vi "line to strings.vi"(11 "line":T1) -> (3 "strings":string[](array[string]))   [LabVIEW 2013, in "EthernetIP editor node.lvclass"]
uses:
  EthernetIP editor node.lvclass
  table line.ctl
  <vilib>/NI/TBM Modules/Ethernet IP/channel/EthernetIP Channel.lvclass
  <vilib>/NI/Tag Bus/tag/tag descriptor.lvclass/tag descriptor.ctl
  <vilib>/NI/TBM Modules/Ethernet IP/channel/EthernetIP Channel.lvclass/EthernetIP Channel.ctl
  <vilib>/NI/Tag Bus Module Framework/channel/TBM channel.lvclass/TBM channel.ctl
  <vilib>/NI/Tag Bus/tag/read tag name.vi
  <vilib>/NI/TBM Modules/Ethernet IP/channel/Read Instance ID.vi
  <vilib>/NI/Tag Bus Module Framework/channel/Read channel classification.vi
  <vilib>/NI/TBM Modules/Ethernet IP/channel/Read byte index.vi
  <vilib>/NI/TBM Modules/Ethernet IP/channel/Read subindex.vi
  <vilib>/NI/Tag Bus/tag/read data type.vi
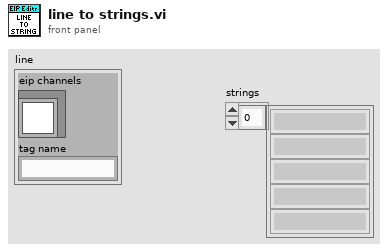
[diagram p1: front panel]
types:
  T1 = typedef "EthernetIP editor node.lvclass/table line.ctl" = cluster{"eip channels":refnum<class "EthernetIP Channel.lvclass">, "tag name":string}
  T2 = typedef "TBM channel.lvclass/channel classification.ctl" = enum16{"input data", "output data", "processing parameter", "processing result"}
  T3 = typedef "tag bus.lvlib/tag descriptor.lvclass/Data Type.ctl" = enum16{"Double", "Single", "I64", "I32", "I16", "I8", "U64", "U32", "U16", "U8", "Boolean", "String", "Array of Double", "Array of Single", "Array of I64", "Array of I32", "Array of I16", "Array of I8", "Array of U64", "Array of U32", "Array of U16", "Array of U8", "Array of Boolean", "Array of String"}
  T4 = typedef "EthernetIP configuration.lvclass/assembly type.ctl" = enum32{"Producing", "Consuming"}
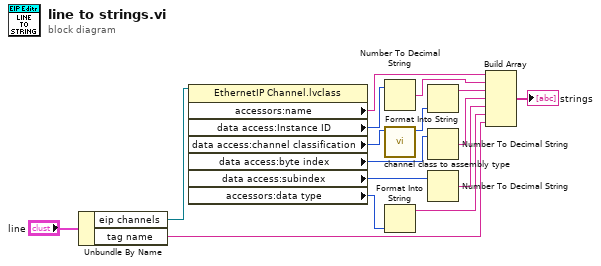
[diagram p0: block diagram]
diagram:
  n1 = Unbundle By Name("line") -> ("eip channels"=w11:refnum<class "EthernetIP Channel.lvclass">, "tag name"=w14:string)
  n2 = property class="EthernetIP Channel.lvclass"(reference=w11) -> ("accessors:name"=w9:string, "data access:Instance ID"=w6:u32, "data access:channel classification"=w8:T2, "data access:byte index"=w4:i32, "data access:subindex"=w3:i32, "accessors:data type"=w10:T3)  [unwired: 1 in, 2 out]
  n3 = Number To Decimal String(number=w6) -> (decimal integer string=w5:string)  [unwired: 1 in]
  n4 = call <vilib>:"channel class to assembly type.vi"("channel classification"=w8) -> ("assembly types"=w7:T4)  [unwired: 10 in]
  n5 = Format Into String(w10) -> (resulting string=w15:string)  [unwired: 3 in, 1 out]
  n6 = Format Into String(w7) -> (resulting string=w12:string)  [unwired: 3 in, 1 out]
  n7 = Number To Decimal String(number=w4) -> (decimal integer string=w1:string)  [unwired: 1 in]
  n8 = Number To Decimal String(number=w3) -> (decimal integer string=w2:string)  [unwired: 1 in]
  n9 = Build Array(w9, w5, w12, w1, w2, w15, w14) -> (→"strings":string[])
